vi "PhotoresistorBoardCounter.vi"() -> ()   [LabVIEW 2018]
uses:
  <vilib>/myRIO/Instrument Drivers/Onboard IO/DIO/typedefs/DIO Reference.ctl
  <vilib>/myRIO/Common/Instrument Driver Framework/Utilities/typedefs/myRIO Generic Hardware Reference.ctl
  <vilib>/myRIO/Common/Instrument Driver Framework/Utilities/typedefs/Hardware Version Enum.ctl
  <vilib>/myRIO/Common/Instrument Driver Framework/Utilities/typedefs/myRIO v1.0 Reference.ctl
  <vilib>/myRIO/Common/Instrument Driver Framework/Utilities/typedefs/Generic FPGA Reference.ctl
  <vilib>/myRIO/Common/Instrument Driver Framework/myRIO v1.0/DIO/typedefs/DIO Channels List.ctl
  <vilib>/myRIO/Common/Instrument Driver Framework/myRIO v1.0/DIO/typedefs/DIO Channels Enum.ctl
  <vilib>/userdefined/High Color/nirio_resource_hc.ctl
  <vilib>/myRIO/Common/Instrument Driver Framework/Utilities/vis/Is FPGA Ref Available.vi
  <vilib>/myRIO/Common/Instrument Driver Framework/myRIO v1.0/DIO/vis/myRIO v1.1 Open DIO.vi
  <vilib>/myRIO/Instrument Drivers/Onboard IO/DIO/vis/Read.vi
  <vilib>/myRIO/Common/Instrument Driver Framework/Utilities/vis/Validate Channels.vi
  <vilib>/myRIO/Common/Instrument Driver Framework/myRIO v1.0/DIO/vis/myRIO v1.0 Reserve DIO.vi
  <vilib>/myRIO/Common/Instrument Driver Framework/myRIO v1.0/Resource Manager/vis/myRIO v1.0 Reserve Channel List.vi
  <vilib>/myRIO/Common/Instrument Driver Framework/myRIO v1.0/DIO/vis/myRIO v1.0 Build MUX Configuration DIO.vi
  <vilib>/myRIO/Common/Instrument Driver Framework/myRIO v1.0/Resource Manager/vis/myRIO v1.0 Reserve Channel.vi
  <vilib>/myRIO/Common/Instrument Driver Framework/myRIO v1.0/Resource Manager/vis/myRIO v1.0 Unreserve Channel.vi
  <vilib>/myRIO/Common/Instrument Driver Framework/myRIO v1.0/Resource Manager/vis/myRIO v1.0 Create Configuration List.vi
  <vilib>/myRIO/Common/Instrument Driver Framework/myRIO v1.0/Resource Manager/vis/myRIO v1.0 Build Mutex Name.vi
  <vilib>/Utility/VariantDataType/GetNumericInfo.vi
  <vilib>/Utility/error.llb/Error Cluster From Error Code.vi
  <vilib>/myRIO/Common/Instrument Driver Framework/myRIO v1.0/myRIO v1.1 Open.vi
  <vilib>/myRIO/Common/Instrument Driver Framework/Utilities/vis/IO Manager.vi
  <vilib>/myRIO/Common/Instrument Driver Framework/Utilities/vis/Configuration Manager.vi
  <vilib>/myRIO/Common/Instrument Driver Framework/myRIO v1.0/Resource Manager/vis/myRIO v1.0 Configure IO.vi
  <vilib>/myRIO/Common/Instrument Driver Framework/myRIO v1.0/myRIO v1.0 Close.vi
  <vilib>/myRIO/Common/Instrument Driver Framework/myRIO v1.0/DIO/vis/myRIO v1.0 Read DIO.vi
  <vilib>/myRIO/Express VI/Onboard IO/DI/DI Express VI.xnode
  <vilib>/myRIO/Instrument Drivers/Onboard IO/DIO/vis/myRIO DIO Open.xnode
  <vilib>/myRIO/Instrument Drivers/Onboard IO/DIO/DIO.lvlib
panel:
  out "output array":i16[](array[numeric])
  out "appended array":bool[](array[boolean])
  in  "stop":bool
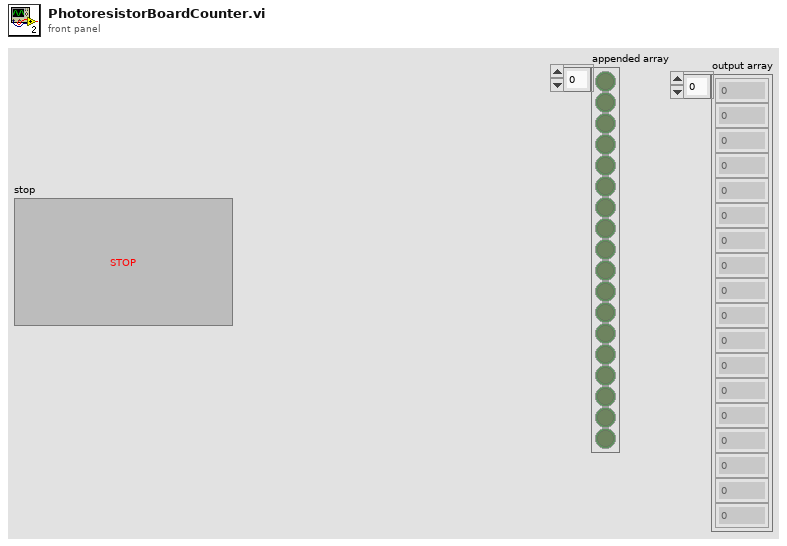
[diagram p1: front panel]
types:
  T1 = typedef "DIO.lvlib/DIO Reference.ctl" = cluster{"myRIO Reference":T2, "DIO Channels List":T6}
  T2 = typedef "myRIO Generic Hardware Reference.ctl" = cluster{"myRIO Model":T3, "myRIO Hardware Reference":T4}
  T3 = typedef "Hardware Version Enum.ctl" = enum16{"Unknown", "myRIO-1900", "myRIO-1950", "roboRIO", "NI ELVIS RIO CM", "ELVIS III"}
  T4 = typedef "myRIO v1.0 Reference.ctl" = cluster{"Generic FPGA Reference":T5, "Allow multiple opens":bool}
  T5 = typedef "Generic FPGA Reference.ctl" = refnum<k20>
  T6 = typedef "DIO Channels List.ctl" = T7[]
  T7 = typedef "DIO Channels Enum.ctl" = enum16{"Not Connected", "C/DIO0", "C/DIO1", "C/DIO2", "C/DIO3", "C/DIO4", "C/DIO5", "C/DIO6", "C/DIO7", "A/DIO0", "A/DIO1", "A/DIO2", "A/DIO3", "A/DIO4", "A/DIO5", "A/DIO6", "A/DIO7", "A/DIO8", "A/DIO9", "A/DIO10", "A/DIO11", "A/DIO12", "A/DIO13", "A/DIO14", "A/DIO15", "A/DIO16", "A/DIO17", "A/DIO18", "A/DIO19", "B/DIO0", "B/DIO1", "B/DIO2", "B/DIO3", "B/DIO4", "B/DIO5", "B/DIO6", "B/DIO7", "B/DIO8", "B/DIO9", "B/DIO10", "B/DIO11", "B/DIO12", "B/DIO13", "B/DIO14", "B/DIO15", "B/DIO16", "B/DIO17", "B/DIO18", "B/DIO19", "LED0", "LED1", "LED2", "LED3", "Button0", "DIO/DIO0", "DIO/DIO1", "DIO/DIO2", "DIO/DIO3", "DIO/DIO4", "DIO/DIO5", "DIO/DIO6", "DIO/DIO7", "DIO/DIO8", "DIO/DIO9", "SPI/CS0", "SPI/CS1", "SPI/CS2", "SPI/CS3", "LED RADIO (Green)", "LED RADIO (Red)", "LED COMM (Green)", "LED COMM (Red)", "LED MODE (Green)", "LED MODE (Red)"}
  T8 = typedef "nirio_resource_hc.ctl" = tag
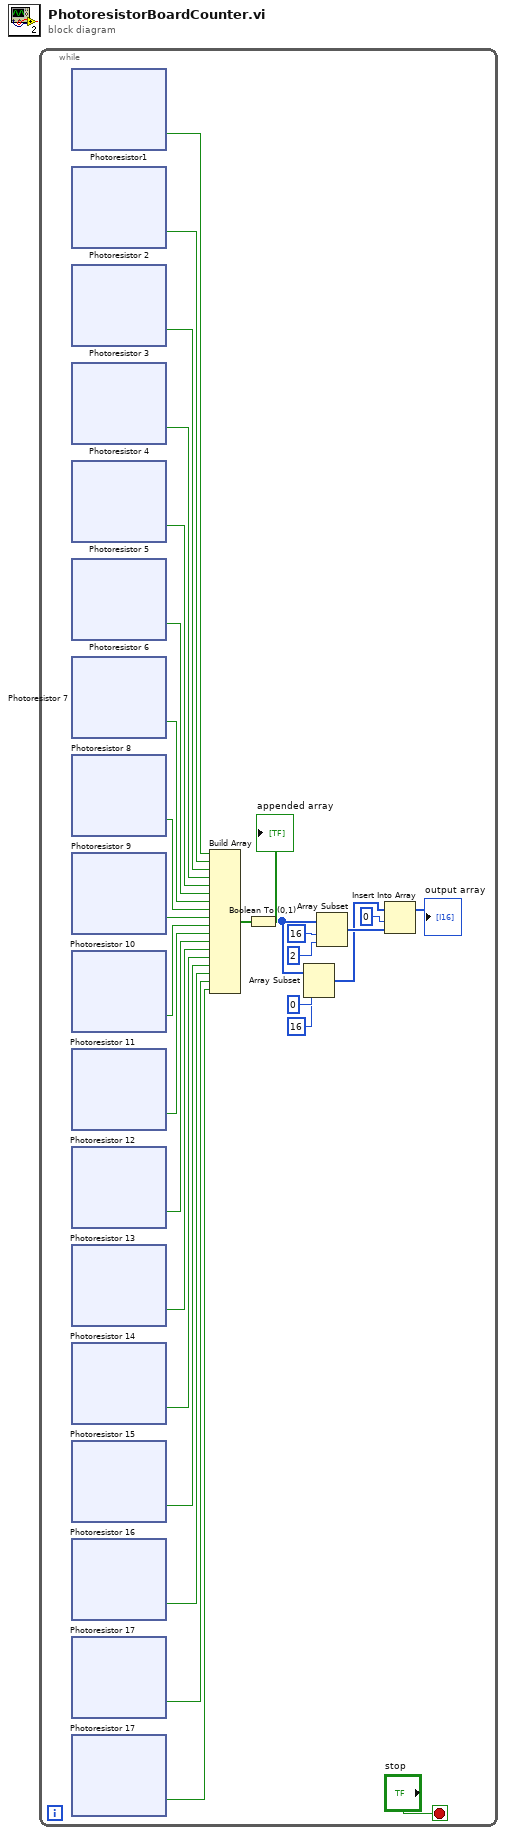
[diagram p0: block diagram]
diagram:
  n1 = while {
    stop <- "stop" stop-if-true
    n2 = xnode "Photoresistor1"() -> ("A/DIO0 (Pin 11)"=w28:bool)  [unwired: 1 in, 1 out]
    n3 = xnode "Photoresistor 2"() -> ("A/DIO1 (Pin 13)"=w27:bool)  [unwired: 1 in, 1 out]
    n4 = xnode "Photoresistor 3"() -> ("A/DIO2 (Pin 15)"=w26:bool)  [unwired: 1 in, 1 out]
    n5 = xnode "Photoresistor 4"() -> ("A/DIO3 (Pin 17)"=w25:bool)  [unwired: 1 in, 1 out]
    n6 = xnode "Photoresistor 5"() -> ("A/DIO4 (Pin 19)"=w24:bool)  [unwired: 1 in, 1 out]
    n7 = xnode "Photoresistor 6"() -> ("A/DIO5 (Pin 21)"=w23:bool)  [unwired: 1 in, 1 out]
    n8 = xnode "Photoresistor 7"() -> ("A/DIO6 (Pin 23)"=w22:bool)  [unwired: 1 in, 1 out]
    n9 = xnode "Photoresistor 8"() -> ("A/DIO7 (Pin 25)"=w21:bool)  [unwired: 1 in, 1 out]
    n10 = xnode "Photoresistor 9"() -> ("A/DIO8 (Pin 27)"=w20:bool)  [unwired: 1 in, 1 out]
    n11 = xnode "Photoresistor 10"() -> ("A/DIO9 (Pin 29)"=w19:bool)  [unwired: 1 in, 1 out]
    n12 = xnode "Photoresistor 11"() -> ("A/DIO10 (Pin 31)"=w18:bool)  [unwired: 1 in, 1 out]
    n13 = xnode "Photoresistor 12"() -> ("A/DIO11 (Pin 18)"=w17:bool)  [unwired: 1 in, 1 out]
    n14 = xnode "Photoresistor 13"() -> ("A/DIO12 (Pin 22)"=w16:bool)  [unwired: 1 in, 1 out]
    n15 = xnode "Photoresistor 14"() -> ("A/DIO13 (Pin 26)"=w15:bool)  [unwired: 1 in, 1 out]
    n16 = xnode "Photoresistor 15"() -> ("A/DIO14 (Pin 32)"=w14:bool)  [unwired: 1 in, 1 out]
    n17 = xnode "Photoresistor 16"() -> ("A/DIO15 (Pin 34)"=w13:bool)  [unwired: 1 in, 1 out]
    n18 = xnode "Photoresistor 17"() -> ("B/DIO14 (Pin 32)"=w11:bool)  [unwired: 1 in, 1 out]
    n19 = xnode "Photoresistor 17"() -> ("B/DIO15 (Pin 34)"=w10:bool)  [unwired: 1 in, 1 out]
    n20 = Build Array(w28, w27, w26, w25, w24, w23, w22, w21, w20, w19, w18, w17, w16, w15, w14, w13, w11, w10) -> (w12:bool[])
    "appended array" <- w12
    n21 = Boolean To (0,1)(Boolean=w12) -> (0, 1=w4:i16[])
    n22 = Array Subset(array=w4, index=0, length=16) -> (w2:i16[])
    n23 = Array Subset(array=w4, index=16, length=2) -> (w5:i16[])
    n24 = Insert Into Array(array=w2, index=0, new element=w5) -> (→"output array":i16[])
  }
